vi "Apply Configuration.vi"(8 "error in (no error)":errorcluster, 11 "IInstrument Base in":refnum<class "IInstrument Base.lvclass">) -> (0 "error out":errorcluster, 3 "IInstrument Base out":refnum<class "IInstrument Base.lvclass">)   [LabVIEW 2023, in "HAL Interfaces.lvlib" / "IInstrument Base.lvclass"]
uses:
  IInstrument Base.lvclass
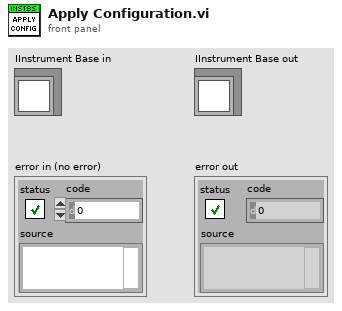
[diagram p1: front panel]
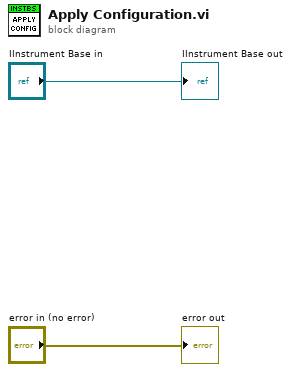
[diagram p0: block diagram]
diagram:
  "error out" <- "error in (no error)"
  "IInstrument Base out" <- "IInstrument Base in"
